vi "Constructor.vi"(8 "ErrorIn":errorcluster, 11 "YAFFooter:YAFFooter in":refnum<class "YAFFooter.lvclass">) -> (0 "ErrorOut":errorcluster, 3 "YAFFooter:YAFFooter out":refnum<class "YAFFooter.lvclass">)   [LabVIEW 2021, in "YAFFooter.lvlib" / "YAFFooter.lvclass"]
uses:
  YAFFooter.lvclass
  YAFFooter.lvclass/YAFFooter.ctl
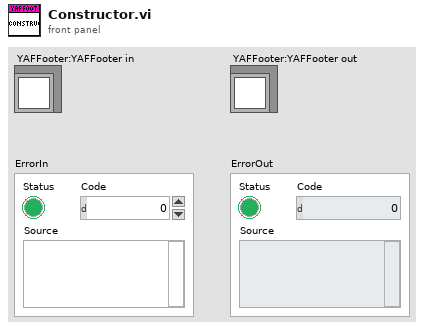
[diagram p1: front panel]
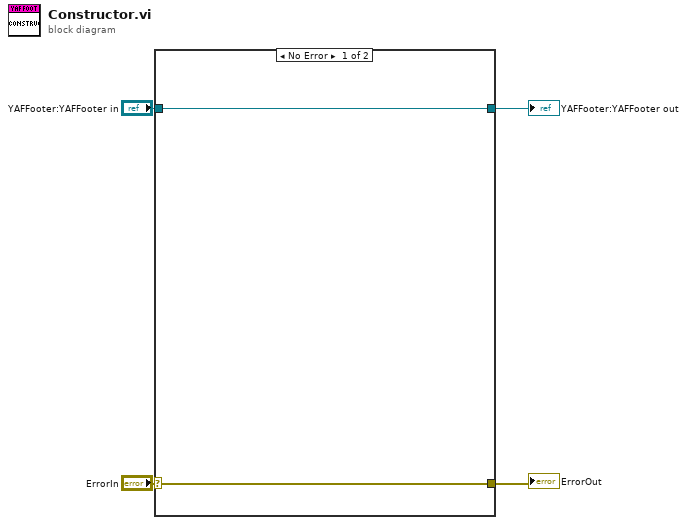
[diagram p0: block diagram]
diagram:
  n1 = case shown="No Error" "ErrorIn" {
    selector: "ErrorIn" -> [w5 w8]
    tunnel: [w5 w8] -> w3
    tunnel: [w6 w7] -> w1
    tunnel: "YAFFooter:YAFFooter in" -> [w6 w7]
    frame No Error {
    }
    frame Error {
    }
  }
  "ErrorOut" <- w3
  "YAFFooter:YAFFooter out" <- w1
